vi "Add New Worker MHLC.vi"(8 "error in (no error)":errorcluster, 10 "Data in":variant, 11 "AppMgr in":refnum<class "Application Manager.lvclass">) -> (0 "error out":errorcluster, 3 "AppMgr out":refnum<class "Application Manager.lvclass">)   [LabVIEW 2017, in "Application Manager.lvclass"]
doc: "A new Worker has been added to the Debug Client. Add to tree and send Response to Caller"
uses:
  Application Manager.lvclass
  C:/Program Files (x86)/National Instruments/LabVIEW 2017/vi.lib/addons/_Workers/Library/Classes/Worker/Worker.lvclass
  <vilib>/addons/_Workers/Library/Classes/Worker/Worker Status.ctl
  <vilib>/addons/_Workers/Library/Classes/Worker/Worker.lvclass/Worker.ctl
  <vilib>/addons/_Workers/Library/Classes/Message/Message.lvclass/Message.ctl
  Application Manager.lvclass/Application Manager.ctl
  Debug Client Data.ctl
  Common VIs/DC_UID.ctl
  Worker Data.ctl
  <vilib>/addons/_Workers/Library/Classes/Worker/Worker Type.ctl
  rsp_New Head Worker Added.ctl
  <vilib>/addons/_Workers/Library/Classes/Worker/Read Message.vi
  <vilib>/addons/_Workers/Library/Classes/Message/Read Sender WID.vi
  Common VIs/DC Name to DC_UID.vi
  <vilib>/addons/_Workers/Library/Classes/Worker/Worker.lvclass
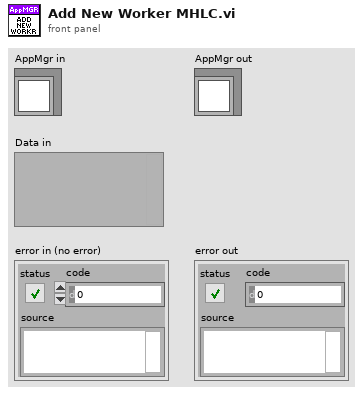
[diagram p1: front panel]
types:
  T1 = typedef "Workers.lvlib/Worker.lvclass/Worker Status.ctl" = enum16{"Queue created", "Preinitialized", "Initialize called", "Initialized", "Start Exiting called", "Exited", "Stopped (Critical Error)"}
  T2 = typedef "DC_UID.ctl" = string
  T3 = typedef "Application Manager.lvclass/Debug Client Data.ctl" = cluster{"DC_UID":T2, "IP Address":string, "Worker Data":T4[], "Connected":bool}
  T4 = typedef "Application Manager.lvclass/Worker Data.ctl" = cluster{"ID":string, "VI Ref":refnum<vi>, "VI Path":path, "CloneID":string, "Type":T5, "Worker Status":string}
  T5 = typedef "Workers.lvlib/Worker.lvclass/Worker Type.ctl" = enum16{"SL", "DL"}
  T6 = typedef "Application Manager.lvclass/rsp_New Head Worker Added.ctl" = cluster{"Head Worker ID":string, "IP Address":string, "DC_UID":T2}
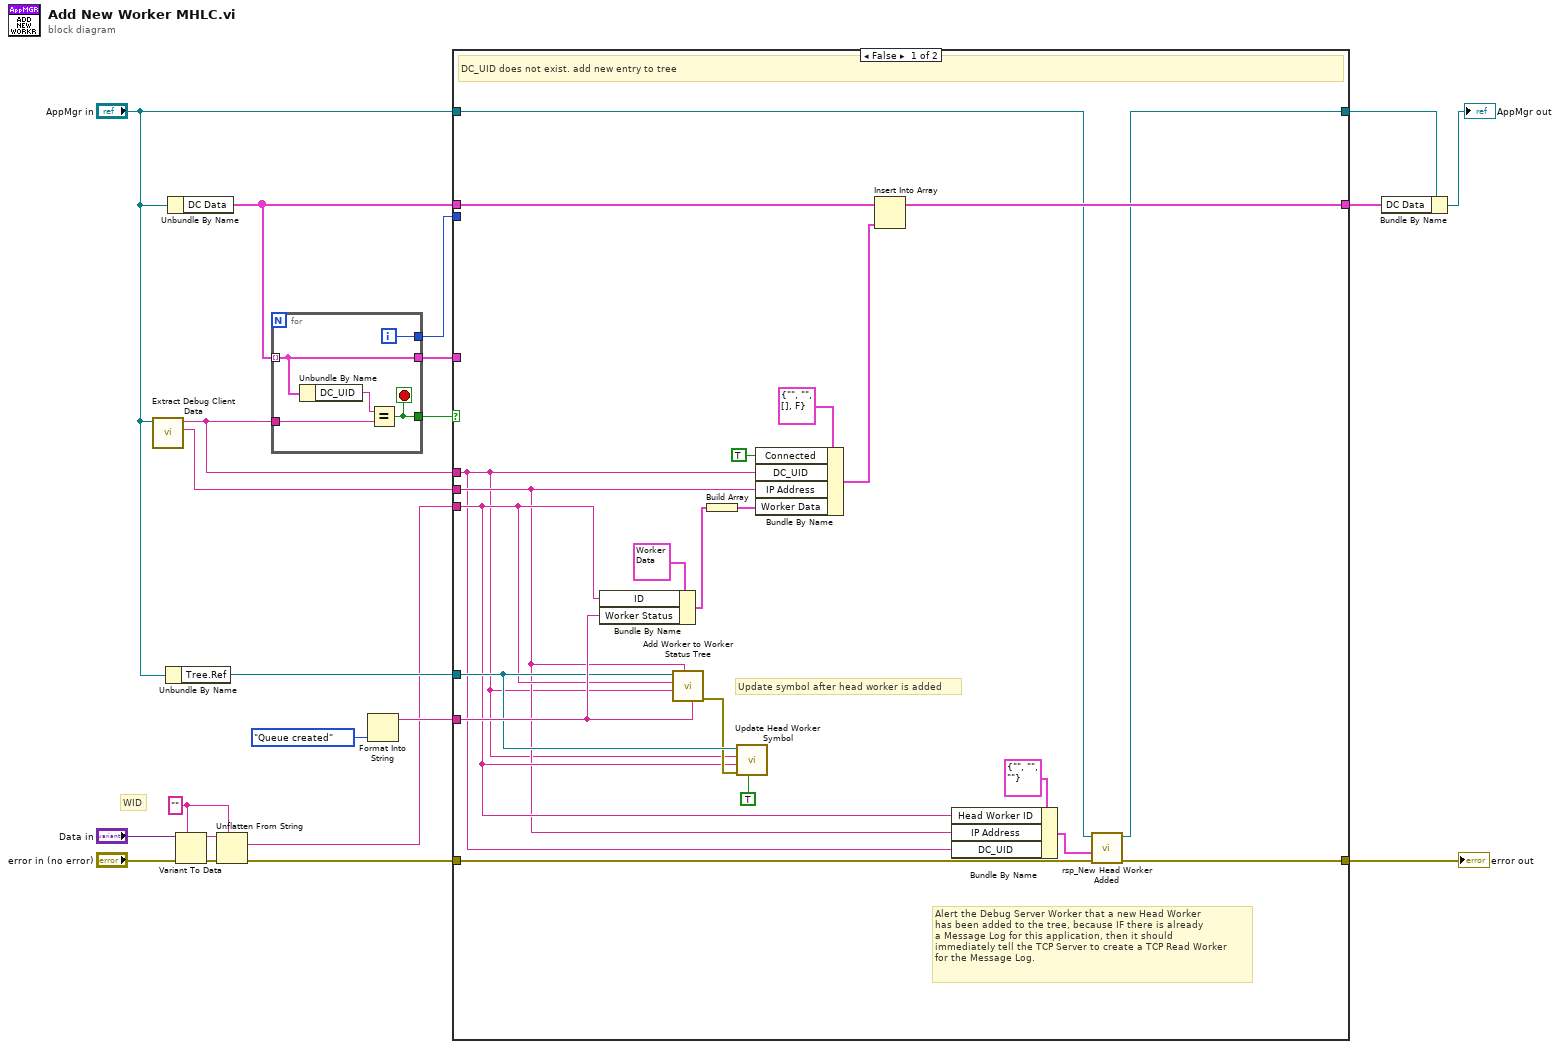
[diagram p0: block diagram]
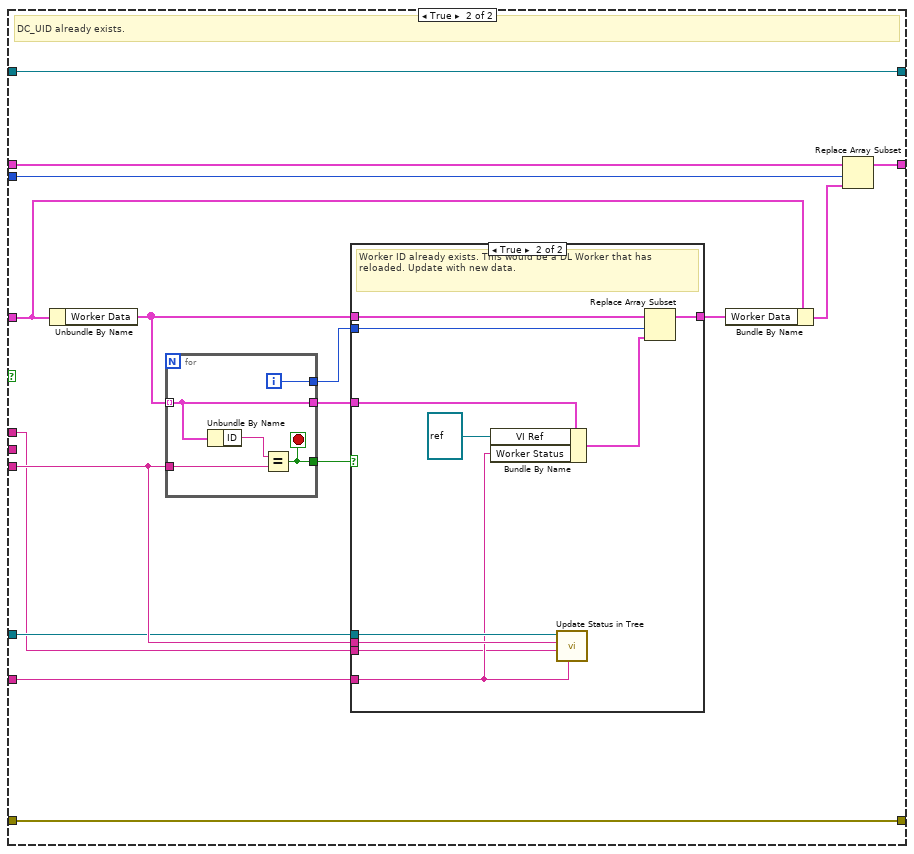
[diagram p2: hidden frame]
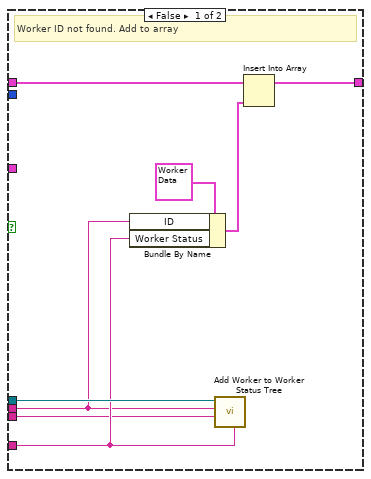
[diagram p3: hidden frame]
diagram:
  w20 = ""
  # "WID"
  n1 = call "Extract Debug Client Data.vi"("AppMgr in"="AppMgr in") -> ("IP Address"=w14:string, "DC_UID"=w15:T2)  [unwired: 9 in]
  n2 = Unbundle By Name("AppMgr in") -> ("Tree.Ref"=w13:refnum<vi>)
  n3 = Unbundle By Name("AppMgr in") -> ("DC Data"=w16:T3[])
  n4 = Variant To Data(error in="error in (no error)", type=w20, Variant="Data in") -> (data=w19:string, error out=w21:errorcluster)
  n5 = Unflatten From String(type=w20, binary string=w19, error in (no error)=w21) -> (value=w3:string, error out=w5:errorcluster)  [unwired: 2 in, 1 out]
  n6 = for {
    tunnel: w16 -> [w22] mode=indexing
    tunnel: w15 -> [w25]
    tunnel: [w24] -> w6
    tunnel: [w23] -> w12
    tunnel: [w22] -> w10
    i -> [w23]
    stop <- w24 stop-if-true
    n7 = Unbundle By Name(w22) -> ("DC_UID"=w26:T2)
    n8 = Equal?(x=w26, y=w25) -> (x = y?=w24:bool)
  }
  n9 = Format Into String(Worker_Status."Queue created" ("Worker Status")) -> (resulting string=w8:string)  [unwired: 3 in, 1 out]
  n10 = case shown="False" w6 {
    tunnel: w16 -> [w42 w63]
    tunnel: w15 -> [w27 w50]
    tunnel: w3 -> [w29 w54]
    tunnel: w14 -> [w28 _]
    tunnel: w13 -> [w38 w51]
    tunnel: w12 -> [_ w61]
    tunnel: [w41 w62] -> w11
    tunnel: w10 -> [_ w59]
    tunnel: w8 -> [w40 w53]
    tunnel: w5 -> [w37 w49]
    tunnel: [w34 w49] -> w4
    tunnel: [w32 w48] -> w2
    tunnel: "AppMgr in" -> [w33 w48]
    frame False {
      # "Alert the Debug Server Worker that a new Head Worker\nhas been added to the tree, because IF there is already\na Message Log for this application, then it should\nimmediately tell the TCP Server to create a TCP Read Worker\nfor the Message Log."
      # "Update symbol after head worker is added"
      # "DC_UID does not exist. add new entry to tree"
      n11 = Bundle By Name(cluster=T4 {"ID"="", "VI Ref"=refnum, "VI Path"=path "", "CloneID"="", "Type"=enum."SL", "Worker Status"=""} ("Worker Data"), "ID"=w29, "Worker Status"=w40) -> (w44:T4)
      n12 = call "Add Worker to Worker Status Tree.vi"("Worker Status"=w40, "IP Address"=w28, "DC_UID"=w27, "WID"=w29, "Tree Ref"=w38) -> ("error out"=w36:errorcluster)  [unwired: 6 in]
      n13 = Build Array(w44) -> (w43:T4[])
      n14 = call "Update Head Worker Symbol.vi"("Connected?"=TRUE, "error in (no error)"=w36, "WID"=w29, "DC_UID"=w27, "Tree Ref"=w38) -> ()  [unwired: 6 in, 1 out]
      n15 = Bundle By Name(cluster=T3 {"DC_UID"="", "IP Address"="", "Worker Data"=[], "Connected"=FALSE} ("DC Data"), "Connected"=TRUE, "DC_UID"=w27, "IP Address"=w28, "Worker Data"=w43) -> (w46:T3)
      n16 = Insert Into Array(array=w42, new element=w46) -> (w41:T3[])  [unwired: 1 in]
      n17 = Bundle By Name(cluster=T6 {"Head Worker ID"="", "IP Address"="", "DC_UID"=""} ("Data in"), "Head Worker ID"=w29, "IP Address"=w28, "DC_UID"=w27) -> (w30:T6)
      n18 = call "rsp_New Head Worker Added.vi"("error in"=w37, "Data in"=w30, "Application Manager in"=w33) -> ("error out"=w34:errorcluster, "dup Application Manager out"=w32:refnum<class "Application Manager.lvclass">)  [unwired: 7 in]
    }
    frame True {
      # "DC_UID already exists."
      n19 = Unbundle By Name(w59) -> ("Worker Data"=w57:T4[])
      n20 = for {
        tunnel: w57 -> [w82] mode=indexing
        tunnel: w54 -> [w85]
        tunnel: [w84] -> w60
        tunnel: [w83] -> w55
        tunnel: [w82] -> w52
        i -> [w83]
        stop <- w84 stop-if-true
        n21 = Unbundle By Name(w82) -> ("ID"=w86:string)
        n22 = Equal?(x=w86, y=w85) -> (x = y?=w84:bool)
      }
      n23 = case shown="True" w60 {
        tunnel: w57 -> [w70 w81]
        tunnel: [w68 w80] -> w56
        tunnel: w55 -> [_ w79]
        tunnel: w54 -> [w64 w74]
        tunnel: w53 -> [w66 w73]
        tunnel: w52 -> [_ w78]
        tunnel: w51 -> [w67 w75]
        tunnel: w50 -> [w65 w72]
        frame False {
          # "Worker ID not found. Add to array"
          n24 = Bundle By Name(cluster=T4 {"ID"="", "VI Ref"=refnum, "VI Path"=path "", "CloneID"="", "Type"=enum."SL", "Worker Status"=""} ("Worker Data"), "ID"=w64, "Worker Status"=w66) -> (w69:T4)
          n25 = call "Add Worker to Worker Status Tree.vi"("Worker Status"=w66, "DC_UID"=w65, "WID"=w64, "Tree Ref"=w67) -> ()  [unwired: 7 in, 1 out]
          n26 = Insert Into Array(array=w70, new element=w69) -> (w68:T4[])  [unwired: 1 in]
        }
        frame True {
          # "Worker ID already exists. This would be a DL Worker that has reloaded. Update with new data."
          n27 = Bundle By Name(cluster=w78, "VI Ref"=refnum<vi> refnum, "Worker Status"=w73) -> (w76:T4)
          n28 = call "Update Status in Tree.vi"("Worker Status"=w73, "DC_UID"=w72, "WID"=w74, "Tree Ref"=w75) -> ()  [unwired: 7 in, 1 out]
          n29 = Replace Array Subset(array=w81, new element=w76, index=w79) -> (w80:T4[])
        }
      }
      n30 = Bundle By Name(cluster=w59, "Worker Data"=w56) -> (w58:T3)
      n31 = Replace Array Subset(array=w63, new element=w58, index=w61) -> (w62:T3[])
    }
  }
  "error out" <- w4
  n32 = Bundle By Name(cluster=w2, "DC Data"=w11) -> (→"AppMgr out":refnum<class "Application Manager.lvclass">)
